vi "2.3.vi"() -> ()   [LabVIEW 2020]
panel:
  out "Thermometer":dbl(slide) scale=0.0..100.0
  out "Tank":dbl(slide) scale=0.0..10.0
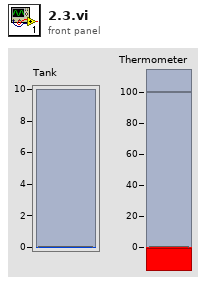
[diagram p1: front panel]
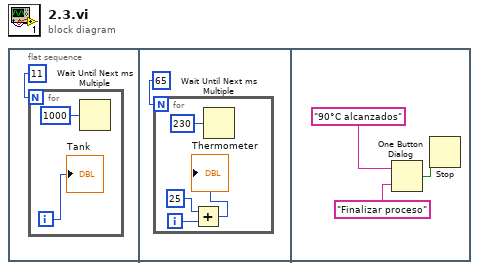
[diagram p0: block diagram]
diagram:
  n1 = flat-sequence {
    frame #0 {
      n2 = for {
        N: 11 -> [_]
        i -> [w2]
        n3 = Wait Until Next ms Multiple(millisecond multiple=u32 1000) -> ()  [unwired: 1 out]
        "Tank" <- w2
      }
    }
    frame #1 {
      n4 = for {
        N: 65 -> [_]
        i -> [w7]
        n5 = Add(x=25, y=w7) -> (x+y=→"Thermometer":i32)
        n6 = Wait Until Next ms Multiple(millisecond multiple=u32 230) -> ()  [unwired: 1 out]
      }
    }
    frame #2 {
      n7 = One Button Dialog(message="90°C alcanzados", button name ("OK")="Finalizar proceso") -> (true=w9:bool)
      n8 = Stop(stop? (T)=w9) -> ()
    }
  }
